vi "Shut Down Device.vi"(8 "error in (no error)":errorcluster, 11 "Coherent Laser Quantum in":refnum<class "Coherent Laser.lvclass">) -> (0 "error out":errorcluster, 3 "Coherent Laser Quantum out":refnum<class "Coherent Laser.lvclass">)   [LabVIEW 2023, in "Coherent Laser.lvlib" / "Coherent Laser.lvclass"]
uses:
  Coherent Laser.lvclass
  Coherent Laser.lvclass/Coherent Laser.ctl
  Laser/Laser.lvclass
  Coherent Laser.lvlib
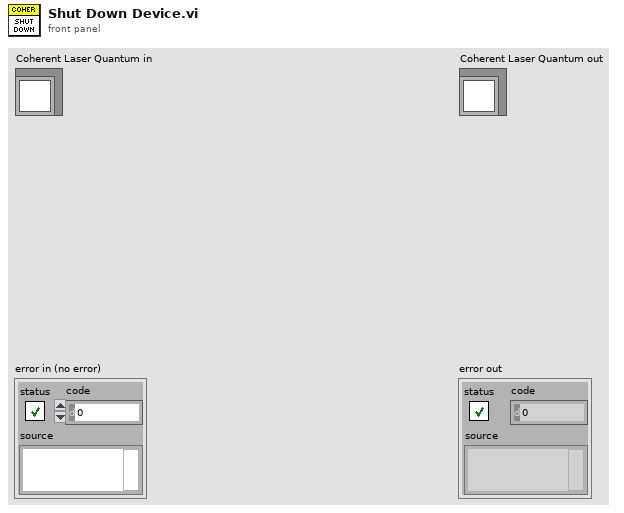
[diagram p1: front panel]
types:
  T1 = enum16{"Disable", "Laser Quantum", "Coherent OBIS", "PRM1-Z8", "Coherent HOPS"}
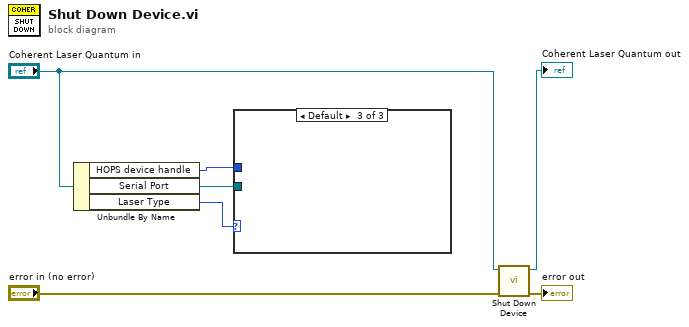
[diagram p0: block diagram]
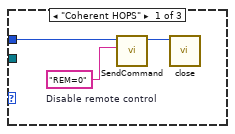
[diagram p2: hidden frame]
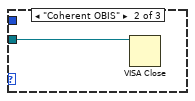
[diagram p3: hidden frame]
diagram:
  n1 = Unbundle By Name("Coherent Laser Quantum in") -> ("HOPS device handle"=w1:u64, "Serial Port"=w4:refnum<visa-resource-name>, "Laser Type"=w3:T1)
  n2 = case shown="Default" w3 {
    tunnel: w4 -> [_ w11 _]
    tunnel: w1 -> [w9 _ _]
    frame "Coherent HOPS" {
      w10 = "REM=0"  # Disable remote control
      n3 = call "SendCommand.vi"("Command"=w10, "Device Handle"=w9) -> ("Dup Handle"=w8:u64)  [unwired: 4 in, 3 out]
      n4 = call "close.vi"("Device Handle"=w8) -> ()  [unwired: 8 in, 1 out]
    }
    frame "Coherent OBIS" {
      n5 = VISA Close(VISA resource name=w11) -> ()  [unwired: 1 in, 1 out]
    }
    frame Default {
    }
  }
  n6 = call-parent "Shut Down Device.vi"("error in (no error)"="error in (no error)", "Device in"="Coherent Laser Quantum in") -> ("error out"=→"error out":errorcluster, "Device out"=→"Coherent Laser Quantum out":refnum<class "Coherent Laser.lvclass">)  [unwired: 8 in]
